vi "Arduino read multiple 11-16-2017 fixed outliers.vi"(10 "arduino addresses in":T2) -> (1 "freq out":dbl[](array[numeric]), 3 "arduino addresses out":T1)   [LabVIEW 2014]
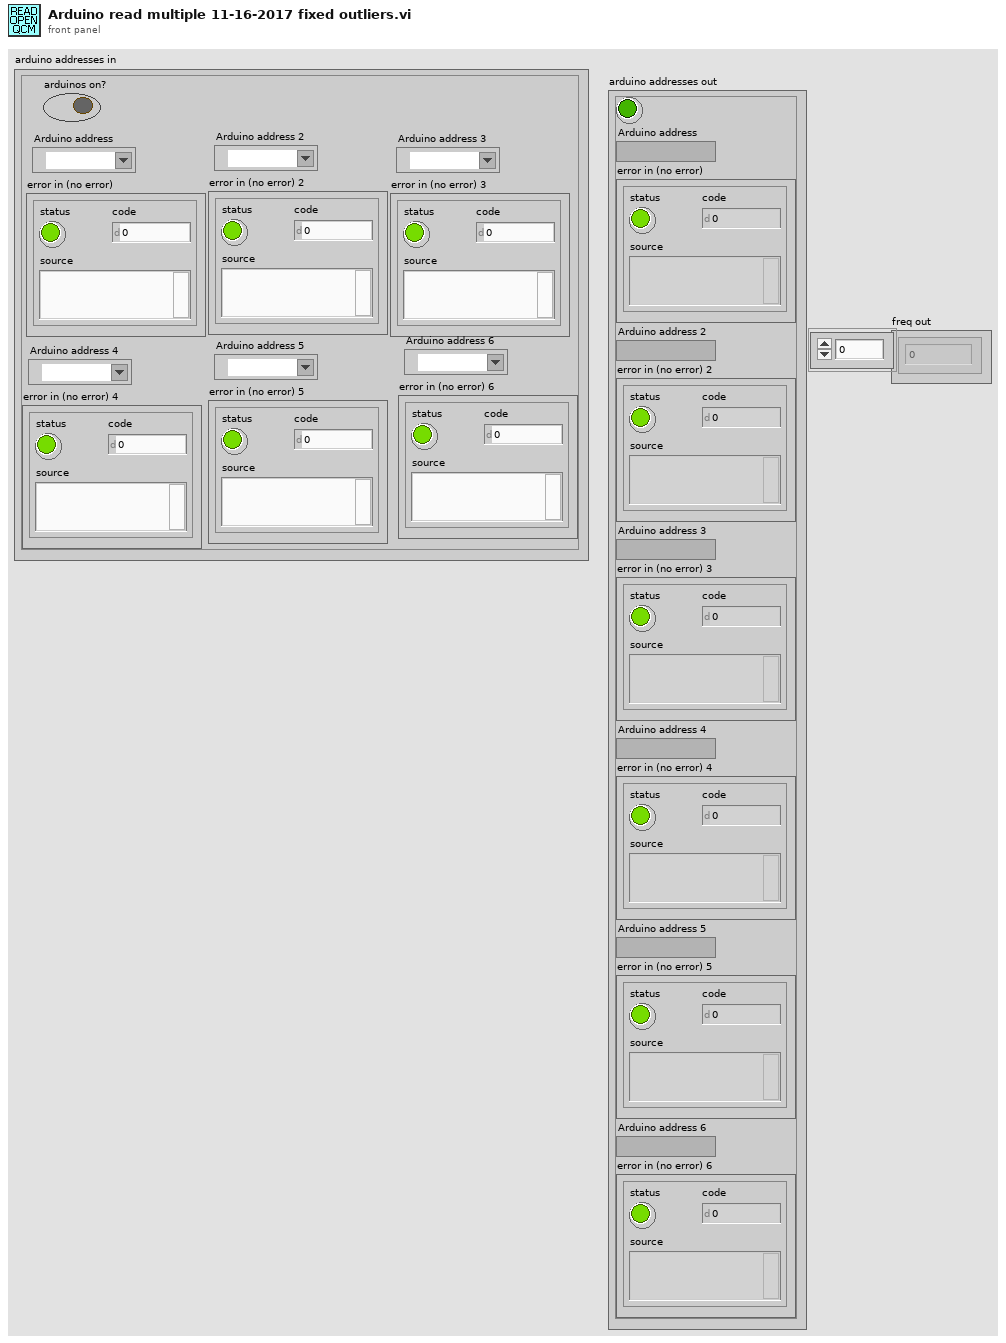
[diagram p1: front panel]
types:
  T1 = cluster{"Boolean":bool, "Arduino address":refnum<visa-resource-name>, "error in (no error)":errorcluster, "Arduino address 2":refnum<visa-resource-name>, "error in (no error) 2":errorcluster, "Arduino address 3":refnum<visa-resource-name>, "error in (no error) 3":errorcluster, "Arduino address 4":refnum<visa-resource-name>, "error in (no error) 4":errorcluster, "Arduino address 5":refnum<visa-resource-name>, "error in (no error) 5":errorcluster, "Arduino address 6":refnum<visa-resource-name>, "error in (no error) 6":errorcluster}
  T2 = cluster{"Arduino address":refnum<visa-resource-name>, "error in (no error)":errorcluster, "Arduino address 2":refnum<visa-resource-name>, "error in (no error) 2":errorcluster, "Arduino address 3":refnum<visa-resource-name>, "error in (no error) 3":errorcluster, "Arduino address 4":refnum<visa-resource-name>, "error in (no error) 4":errorcluster, "Arduino address 5":refnum<visa-resource-name>, "error in (no error) 5":errorcluster, "Arduino address 6":refnum<visa-resource-name>, "error in (no error) 6":errorcluster, "arduinos on?":bool}
  T3 = cluster{bool, "Arduino address":refnum<visa-resource-name>, "error in (no error)":errorcluster, "Arduino address 2":refnum<visa-resource-name>, "error in (no error) 2":errorcluster, "Arduino address 3":refnum<visa-resource-name>, "error in (no error) 3":errorcluster, "Arduino address 4":refnum<visa-resource-name>, "error in (no error) 4":errorcluster, "Arduino address 5":refnum<visa-resource-name>, "error in (no error) 5":errorcluster, "Arduino address 6":refnum<visa-resource-name>, "error in (no error) 6":errorcluster}
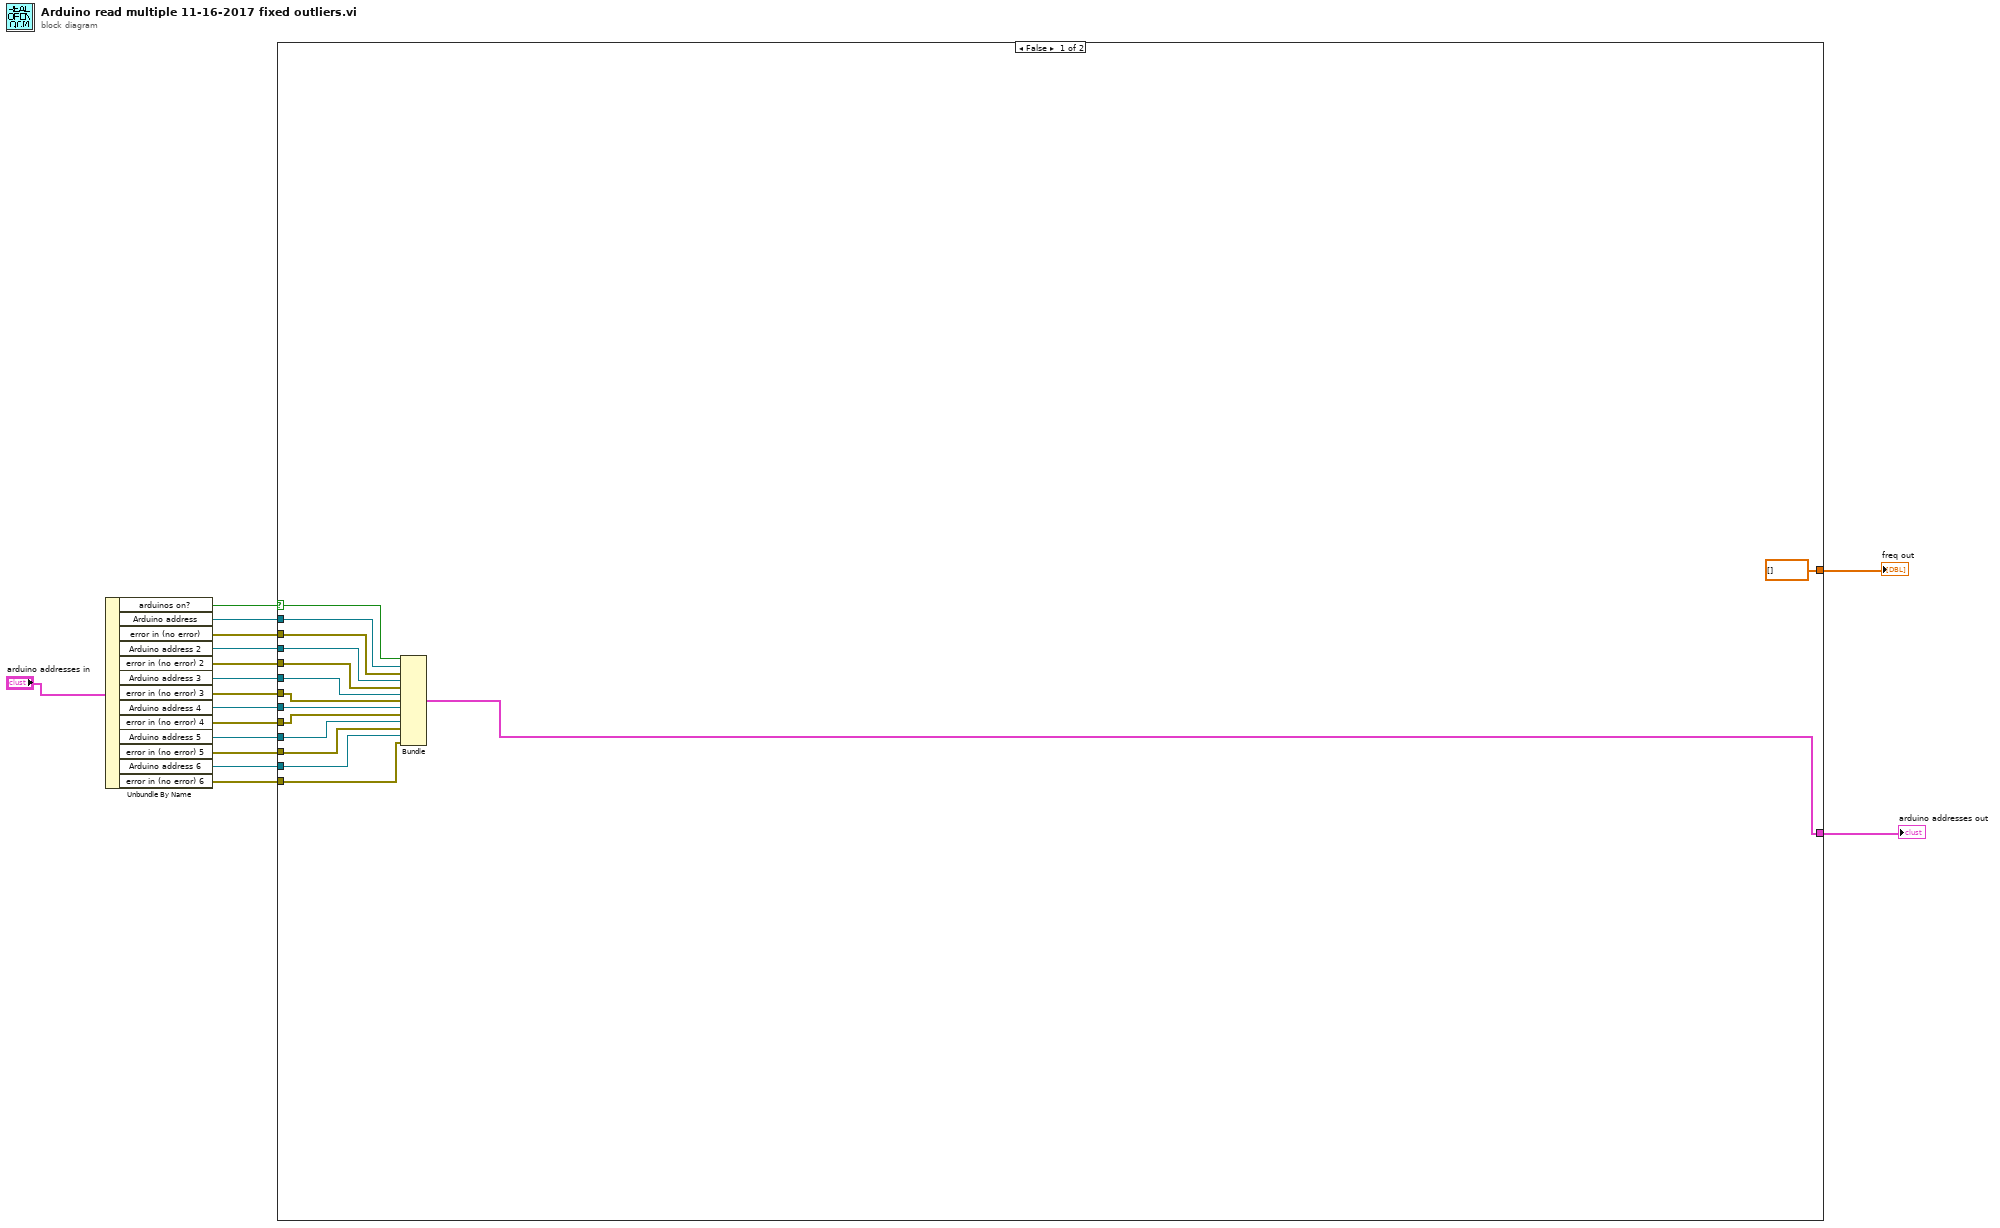
[diagram p0: block diagram]
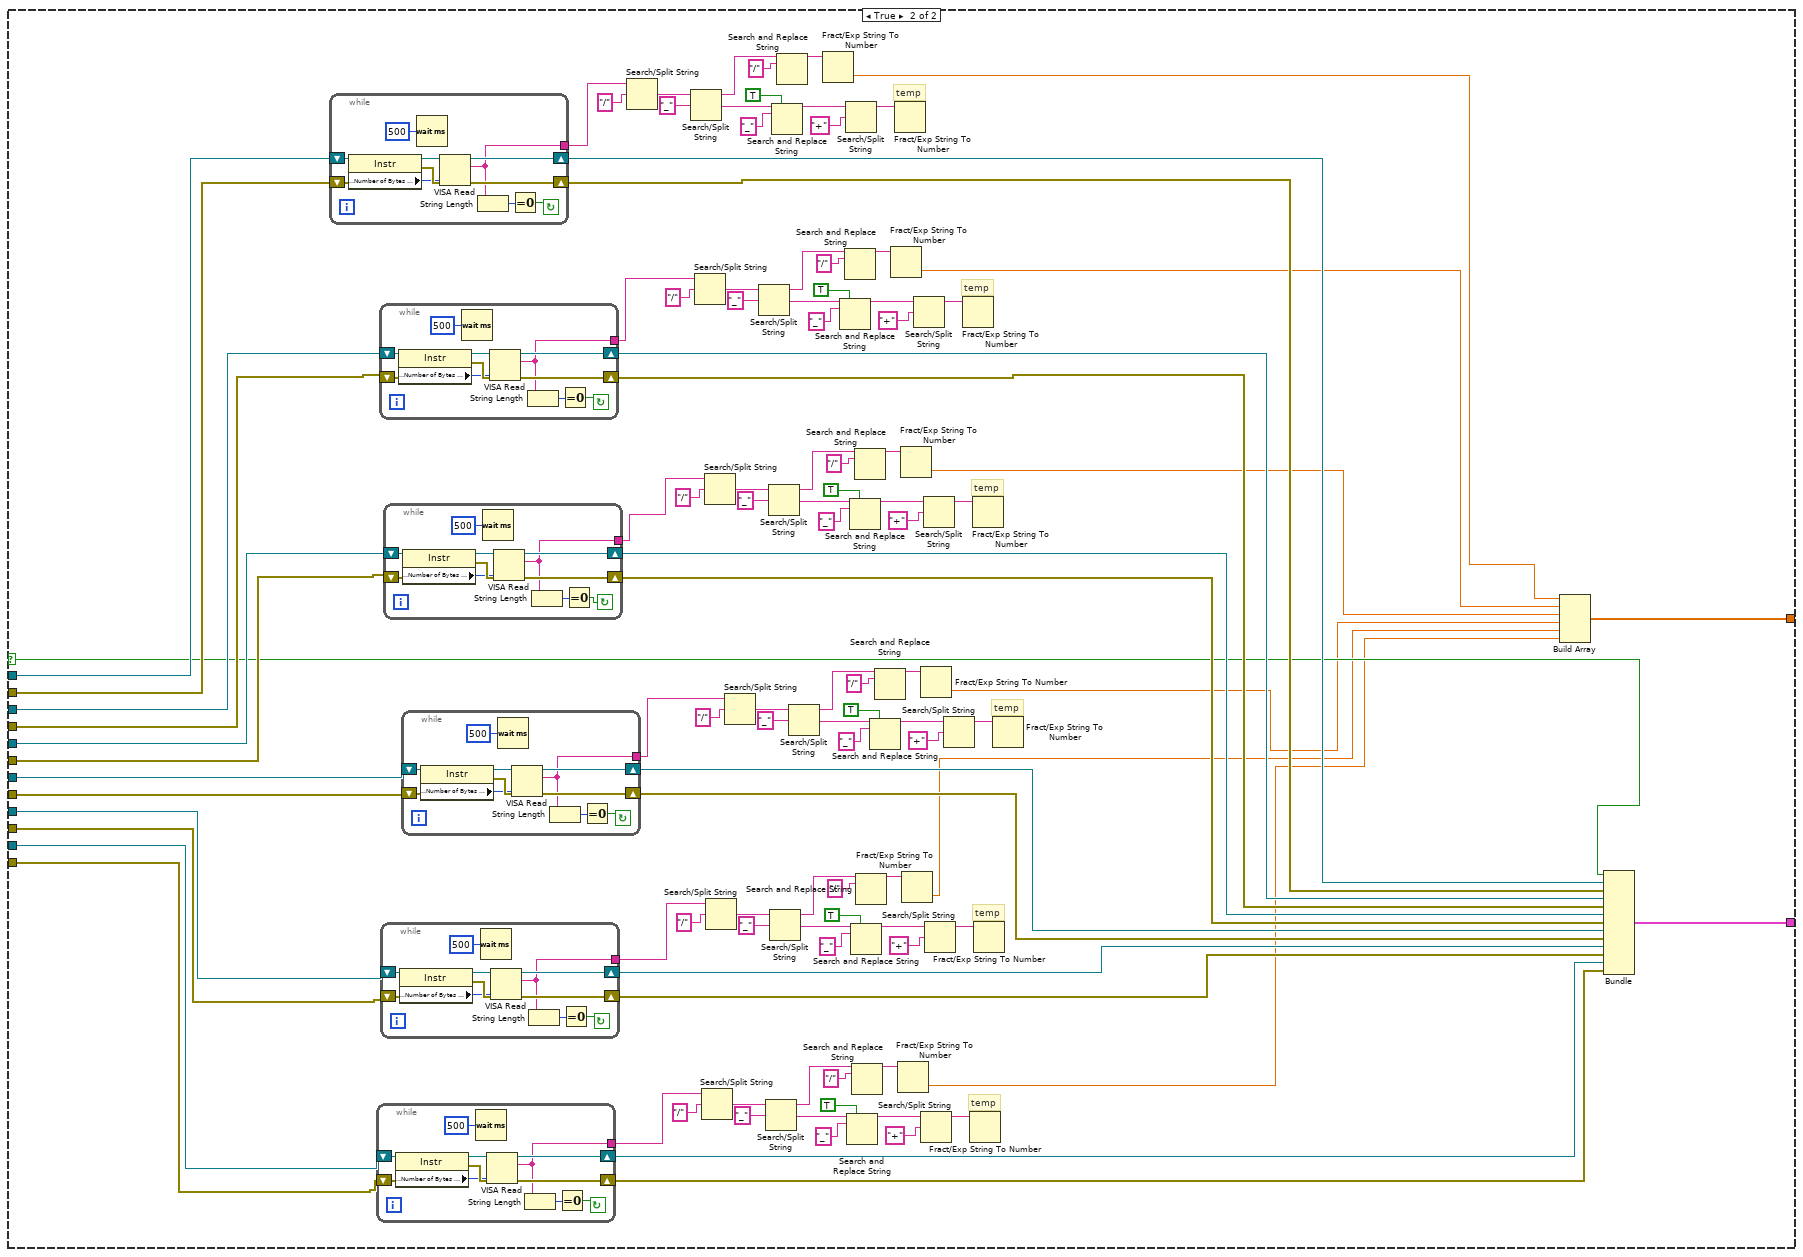
[diagram p2: hidden frame]
diagram:
  n1 = Unbundle By Name("arduino addresses in") -> ("arduinos on?"=w16:bool, "Arduino address"=w15:refnum<visa-resource-name>, "error in (no error)"=w14:errorcluster, "Arduino address 2"=w13:refnum<visa-resource-name>, "error in (no error) 2"=w12:errorcluster, "Arduino address 3"=w11:refnum<visa-resource-name>, "error in (no error) 3"=w10:errorcluster, "Arduino address 4"=w8:refnum<visa-resource-name>, "error in (no error) 4"=w7:errorcluster, "Arduino address 5"=w6:refnum<visa-resource-name>, "error in (no error) 5"=w5:errorcluster, "Arduino address 6"=w4:refnum<visa-resource-name>, "error in (no error) 6"=w3:errorcluster)
  n2 = case shown="False" w16 {
    selector: w16 -> [w31 w40]
    tunnel: [w18 w39] -> w2
    tunnel: w15 -> [w30 w52]
    tunnel: w14 -> [w29 w51]
    tunnel: w13 -> [w28 w50]
    tunnel: w12 -> [w27 w49]
    tunnel: w11 -> [w26 w48]
    tunnel: w10 -> [w25 w47]
    tunnel: w8 -> [w24 w46]
    tunnel: w7 -> [w23 w45]
    tunnel: w6 -> [w22 w44]
    tunnel: w5 -> [w21 w43]
    tunnel: w4 -> [w20 w42]
    tunnel: w3 -> [w19 w41]
    tunnel: [dbl[] [] w32] -> w1
    frame False {
      n3 = Bundle(w31, "Arduino address"=w30, "error in (no error)"=w29, "Arduino address 2"=w28, "error in (no error) 2"=w27, "Arduino address 3"=w26, "error in (no error) 3"=w25, "Arduino address 4"=w24, "error in (no error) 4"=w23, "Arduino address 5"=w22, "error in (no error) 5"=w21, "Arduino address 6"=w20, "error in (no error) 6"=w19) -> (w18:T3)  [unwired: 1 in]
    }
    frame True {
      # "temp"
      # "temp"
      # "temp"
      # "temp"
      # "temp"
      # "temp"
      n4 = while {
        shift-right: [w208] -> w64
        shift-left: w52 -> [w206]
        shift-right: [w207] -> w63
        shift-left: w51 -> [w205]
        tunnel: [w199] -> w130
        stop <- w200 continue-if-true
        n5 = property class="Instr"(reference=w206, error in=w205) -> (reference out=w203:refnum<visa-resource-name>, error out=w204:errorcluster, "Serial Settings:Number of Bytes at Serial Port"=w202:u32)
        n6 = Wait (ms)(milliseconds to wait=u32 500) -> ()  [unwired: 1 out]
        n7 = VISA Read(VISA resource name=w203, byte count=w202, error in (no error)=w204) -> (VISA resource name out=w208:refnum<visa-resource-name>, read buffer=w199:string, error out=w207:errorcluster)  [unwired: 1 out]
        n8 = String Length(string=w199) -> (length=w201:i32)
        n9 = Equal To 0?(x=w201) -> (x = 0?=w200:bool)
      }
      n10 = while {
        shift-right: [w153] -> w55
        shift-left: w42 -> [w151]
        shift-right: [w152] -> w54
        shift-left: w41 -> [w150]
        tunnel: [w144] -> w65
        stop <- w145 continue-if-true
        n11 = property class="Instr"(reference=w151, error in=w150) -> (reference out=w148:refnum<visa-resource-name>, error out=w149:errorcluster, "Serial Settings:Number of Bytes at Serial Port"=w147:u32)
        n12 = Wait (ms)(milliseconds to wait=u32 500) -> ()  [unwired: 1 out]
        n13 = VISA Read(VISA resource name=w148, byte count=w147, error in (no error)=w149) -> (VISA resource name out=w153:refnum<visa-resource-name>, read buffer=w144:string, error out=w152:errorcluster)  [unwired: 1 out]
        n14 = String Length(string=w144) -> (length=w146:i32)
        n15 = Equal To 0?(x=w146) -> (x = 0?=w145:bool)
      }
      n16 = while {
        shift-right: [w197] -> w62
        shift-left: w50 -> [w195]
        shift-right: [w196] -> w61
        shift-left: w49 -> [w194]
        tunnel: [w188] -> w117
        stop <- w189 continue-if-true
        n17 = property class="Instr"(reference=w195, error in=w194) -> (reference out=w192:refnum<visa-resource-name>, error out=w193:errorcluster, "Serial Settings:Number of Bytes at Serial Port"=w191:u32)
        n18 = Wait (ms)(milliseconds to wait=u32 500) -> ()  [unwired: 1 out]
        n19 = VISA Read(VISA resource name=w192, byte count=w191, error in (no error)=w193) -> (VISA resource name out=w197:refnum<visa-resource-name>, read buffer=w188:string, error out=w196:errorcluster)  [unwired: 1 out]
        n20 = String Length(string=w188) -> (length=w190:i32)
        n21 = Equal To 0?(x=w190) -> (x = 0?=w189:bool)
      }
      n22 = while {
        shift-right: [w164] -> w53
        shift-left: w44 -> [w162]
        shift-right: [w163] -> w56
        shift-left: w43 -> [w161]
        tunnel: [w155] -> w78
        stop <- w156 continue-if-true
        n23 = property class="Instr"(reference=w162, error in=w161) -> (reference out=w159:refnum<visa-resource-name>, error out=w160:errorcluster, "Serial Settings:Number of Bytes at Serial Port"=w158:u32)
        n24 = Wait (ms)(milliseconds to wait=u32 500) -> ()  [unwired: 1 out]
        n25 = VISA Read(VISA resource name=w159, byte count=w158, error in (no error)=w160) -> (VISA resource name out=w164:refnum<visa-resource-name>, read buffer=w155:string, error out=w163:errorcluster)  [unwired: 1 out]
        n26 = String Length(string=w155) -> (length=w157:i32)
        n27 = Equal To 0?(x=w157) -> (x = 0?=w156:bool)
      }
      n28 = while {
        shift-right: [w186] -> w60
        shift-left: w48 -> [w184]
        shift-right: [w185] -> w59
        shift-left: w47 -> [w183]
        tunnel: [w177] -> w104
        stop <- w178 continue-if-true
        n29 = property class="Instr"(reference=w184, error in=w183) -> (reference out=w181:refnum<visa-resource-name>, error out=w182:errorcluster, "Serial Settings:Number of Bytes at Serial Port"=w180:u32)
        n30 = Wait (ms)(milliseconds to wait=u32 500) -> ()  [unwired: 1 out]
        n31 = VISA Read(VISA resource name=w181, byte count=w180, error in (no error)=w182) -> (VISA resource name out=w186:refnum<visa-resource-name>, read buffer=w177:string, error out=w185:errorcluster)  [unwired: 1 out]
        n32 = String Length(string=w177) -> (length=w179:i32)
        n33 = Equal To 0?(x=w179) -> (x = 0?=w178:bool)
      }
      n34 = while {
        shift-right: [w175] -> w58
        shift-left: w46 -> [w173]
        shift-right: [w174] -> w57
        shift-left: w45 -> [w172]
        tunnel: [w166] -> w91
        stop <- w167 continue-if-true
        n35 = property class="Instr"(reference=w173, error in=w172) -> (reference out=w170:refnum<visa-resource-name>, error out=w171:errorcluster, "Serial Settings:Number of Bytes at Serial Port"=w169:u32)
        n36 = Wait (ms)(milliseconds to wait=u32 500) -> ()  [unwired: 1 out]
        n37 = VISA Read(VISA resource name=w170, byte count=w169, error in (no error)=w171) -> (VISA resource name out=w175:refnum<visa-resource-name>, read buffer=w166:string, error out=w174:errorcluster)  [unwired: 1 out]
        n38 = String Length(string=w166) -> (length=w168:i32)
        n39 = Equal To 0?(x=w168) -> (x = 0?=w167:bool)
      }
      n40 = Search/Split String(string=w130, search string/char (-)="/") -> (match + rest of string=w136:string)  [unwired: 1 in, 2 out]
      n41 = Search/Split String(string=w136, search string/char (-)="_") -> (substring before match=w142:string, match + rest of string=w137:string)  [unwired: 1 in, 1 out]
      n42 = Search/Split String(string=w117, search string/char (-)="/") -> (match + rest of string=w123:string)  [unwired: 1 in, 2 out]
      n43 = Search/Split String(string=w65, search string/char (-)="/") -> (match + rest of string=w71:string)  [unwired: 1 in, 2 out]
      n44 = Search/Split String(string=w104, search string/char (-)="/") -> (match + rest of string=w110:string)  [unwired: 1 in, 2 out]
      n45 = Search/Split String(string=w78, search string/char (-)="/") -> (match + rest of string=w84:string)  [unwired: 1 in, 2 out]
      n46 = Search/Split String(string=w91, search string/char (-)="/") -> (match + rest of string=w97:string)  [unwired: 1 in, 2 out]
      n47 = Search/Split String(string=w123, search string/char (-)="_") -> (substring before match=w129:string, match + rest of string=w124:string)  [unwired: 1 in, 1 out]
      n48 = Search/Split String(string=w71, search string/char (-)="_") -> (substring before match=w77:string, match + rest of string=w72:string)  [unwired: 1 in, 1 out]
      n49 = Search/Split String(string=w110, search string/char (-)="_") -> (substring before match=w116:string, match + rest of string=w111:string)  [unwired: 1 in, 1 out]
      n50 = Search/Split String(string=w84, search string/char (-)="_") -> (substring before match=w90:string, match + rest of string=w85:string)  [unwired: 1 in, 1 out]
      n51 = Search and Replace String(replace all?=TRUE ("replace all? (F)"), input string=w137, search string="_") -> (result string=w131:string)  [unwired: 5 in, 3 out]
      n52 = Search and Replace String(input string=w142, search string="/" ("replace string (\"\")")) -> (result string=w133:string)  [unwired: 6 in, 3 out]
      n53 = Search/Split String(string=w97, search string/char (-)="_") -> (substring before match=w103:string, match + rest of string=w98:string)  [unwired: 1 in, 1 out]
      n54 = Fract/Exp String To Number(string=w133) -> (number=w38:dbl)  [unwired: 3 in, 1 out]
      n55 = Search and Replace String(replace all?=TRUE ("replace all? (F)"), input string=w124, search string="_") -> (result string=w118:string)  [unwired: 5 in, 3 out]
      n56 = Search and Replace String(input string=w129, search string="/" ("replace string (\"\")")) -> (result string=w120:string)  [unwired: 6 in, 3 out]
      n57 = Search/Split String(string=w131, search string/char (-)="+") -> (substring before match=w140:string)  [unwired: 1 in, 2 out]
      n58 = Search and Replace String(replace all?=TRUE ("replace all? (F)"), input string=w72, search string="_") -> (result string=w66:string)  [unwired: 5 in, 3 out]
      n59 = Search and Replace String(replace all?=TRUE ("replace all? (F)"), input string=w111, search string="_") -> (result string=w105:string)  [unwired: 5 in, 3 out]
      n60 = Search and Replace String(replace all?=TRUE ("replace all? (F)"), input string=w85, search string="_") -> (result string=w79:string)  [unwired: 5 in, 3 out]
      n61 = Search and Replace String(input string=w77, search string="/" ("replace string (\"\")")) -> (result string=w68:string)  [unwired: 6 in, 3 out]
      n62 = Search and Replace String(input string=w116, search string="/" ("replace string (\"\")")) -> (result string=w107:string)  [unwired: 6 in, 3 out]
      n63 = Search and Replace String(input string=w90, search string="/" ("replace string (\"\")")) -> (result string=w81:string)  [unwired: 6 in, 3 out]
      n64 = Search and Replace String(replace all?=TRUE ("replace all? (F)"), input string=w98, search string="_") -> (result string=w92:string)  [unwired: 5 in, 3 out]
      n65 = Search and Replace String(input string=w103, search string="/" ("replace string (\"\")")) -> (result string=w94:string)  [unwired: 6 in, 3 out]
      n66 = Fract/Exp String To Number(string=w120) -> (number=w37:dbl)  [unwired: 3 in, 1 out]
      n67 = Fract/Exp String To Number(string=w140) -> ()  [unwired: 3 in, 2 out]
      n68 = Fract/Exp String To Number(string=w68) -> (number=w33:dbl)  [unwired: 3 in, 1 out]
      n69 = Fract/Exp String To Number(string=w107) -> (number=w36:dbl)  [unwired: 3 in, 1 out]
      n70 = Fract/Exp String To Number(string=w81) -> (number=w34:dbl)  [unwired: 3 in, 1 out]
      n71 = Search/Split String(string=w118, search string/char (-)="+") -> (substring before match=w127:string)  [unwired: 1 in, 2 out]
      n72 = Fract/Exp String To Number(string=w94) -> (number=w35:dbl)  [unwired: 3 in, 1 out]
      n73 = Search/Split String(string=w66, search string/char (-)="+") -> (substring before match=w75:string)  [unwired: 1 in, 2 out]
      n74 = Search/Split String(string=w105, search string/char (-)="+") -> (substring before match=w114:string)  [unwired: 1 in, 2 out]
      n75 = Search/Split String(string=w79, search string/char (-)="+") -> (substring before match=w88:string)  [unwired: 1 in, 2 out]
      n76 = Search/Split String(string=w92, search string/char (-)="+") -> (substring before match=w101:string)  [unwired: 1 in, 2 out]
      n77 = Fract/Exp String To Number(string=w127) -> ()  [unwired: 3 in, 2 out]
      n78 = Fract/Exp String To Number(string=w75) -> ()  [unwired: 3 in, 2 out]
      n79 = Fract/Exp String To Number(string=w114) -> ()  [unwired: 3 in, 2 out]
      n80 = Fract/Exp String To Number(string=w88) -> ()  [unwired: 3 in, 2 out]
      n81 = Fract/Exp String To Number(string=w101) -> ()  [unwired: 3 in, 2 out]
      n82 = Build Array(w38, w37, w36, w35, w34, w33) -> (w32:dbl[])
      n83 = Bundle(w40, "Arduino address"=w64, "error in (no error)"=w63, "Arduino address 2"=w62, "error in (no error) 2"=w61, "Arduino address 3"=w60, "error in (no error) 3"=w59, "Arduino address 4"=w58, "error in (no error) 4"=w57, "Arduino address 5"=w53, "error in (no error) 5"=w56, "Arduino address 6"=w55, "error in (no error) 6"=w54) -> (w39:T3)  [unwired: 1 in]
    }
  }
  "arduino addresses out" <- w2
  "freq out" <- w1
